vi "Compare Dependency Sets.vi"(8 "error in (no error)":errorcluster, 10 "Scanned":set{string}(c389) caption="Scanned Dependencies", 11 "Builder in":refnum<class "Builder.lvclass">) -> (0 "error out":errorcluster, 3 "Builder out":refnum<class "Builder.lvclass">)   [LabVIEW 2019, in "Builder.lvclass"]
uses:
  Builder.lvclass
  Builder.lvclass/Builder.ctl
  8787f5ba-6225-4483-b00e-ce340b9170cf.vi
  f372c00e-bb7a-4085-9e1c-f3356340c9e9.vi
  <vilib>/Utility/error.llb/Error Cluster From Error Code.vi
  <vilib>/ErrorRing/Error Ring.xnode
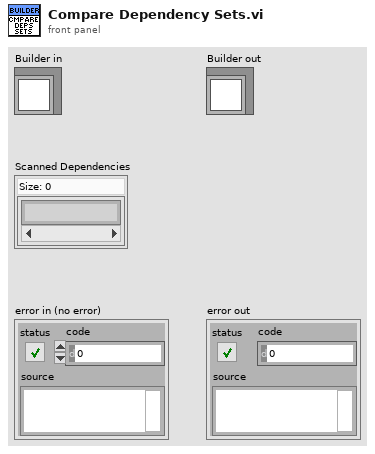
[diagram p1: front panel]
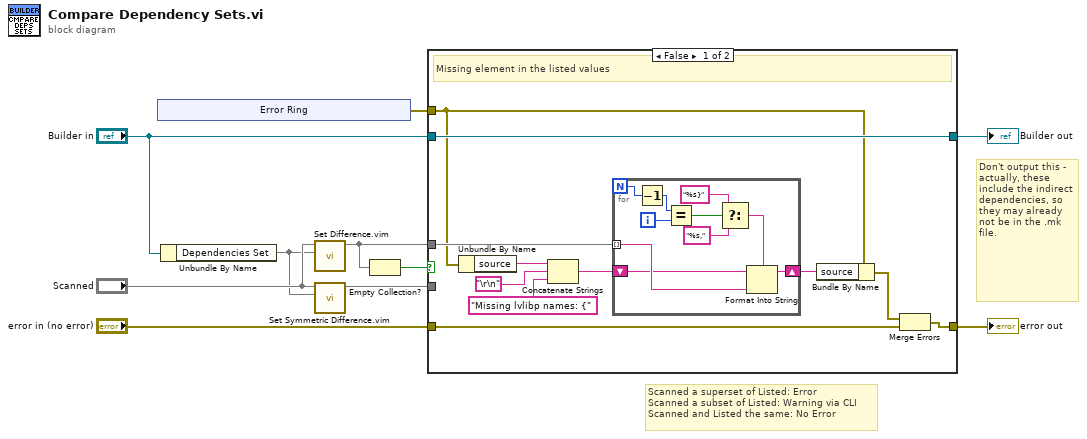
[diagram p0: block diagram]
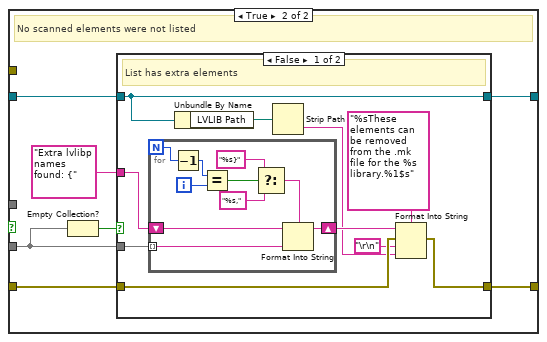
[diagram p2: hidden frame]
diagram:
  # "Don't output this - actually, these include the indirect dependencies, so they may already not be in the .mk file."
  # "Scanned a superset of Listed: Error\nScanned a subset of Listed: Warning via CLI\nScanned and Listed the same: No Error"
  n1 = xnode "Error Ring"() -> ("error out"=w1:errorcluster)
  n2 = Unbundle By Name("Builder in") -> ("Dependencies Set"=w2:set{string})
  n3 = call "Set Difference.vim"("set 2"=w2, "set 1"="Scanned") -> ("difference"=w6:set{string})  [unwired: 9 in]
  n4 = call "Set Symmetric Difference.vim"("set 2"=w2, "set 1"="Scanned") -> ("symmetric difference"=w9:set{string})  [unwired: 9 in]
  n5 = Empty Collection?(1:w6) -> (0:w4:bool)
  n6 = case shown="False" w4 {
    tunnel: w6 -> [w21 _]
    tunnel: "error in (no error)" -> [w20 w33]
    tunnel: [w19 w34] -> w8
    tunnel: w9 -> [_ w35]
    tunnel: "Builder in" -> [w18 w37]
    tunnel: [w18 w36] -> w10
    tunnel: w1 -> [w17 _]
    frame False {
      # "Missing element in the listed values"
      n7 = Unbundle By Name(w17) -> ("source"=w16:string)
      n8 = Concatenate Strings(w16, "\r\n", "Missing lvlibp names: {" ("string")) -> (w15:string)
      n9 = for {
        N -> [w28]
        tunnel: w21 -> [w31] mode=indexing
        shift-right: [w29] -> w11
        shift-left: w15 -> [w30]
        i -> [w26]
        n10 = Decrement(x=w28) -> (x-1=w27:i32)
        n11 = Equal?(x=w27, y=w26) -> (x = y?=w25:bool)
        n12 = Select(t="%s}", s=w25, f="%s,") -> (s? t:f=w22:string)
        n13 = Format Into String(format string=w22, initial string=w30, w31) -> (resulting string=w29:string)  [unwired: 1 in, 1 out]
      }
      n14 = Bundle By Name(cluster=w17, "source"=w11) -> (w12:errorcluster)
      n15 = Merge Errors(w12, w20) -> (w19:errorcluster)
    }
    frame True {
      # "No scanned elements were not listed"
      n16 = Empty Collection?(1:w35) -> (0:w38:bool)
      n17 = case shown="False" w38 {
        tunnel: w37 -> [w46 w60]
        tunnel: [w46 w60] -> w36
        tunnel: w35 -> [w47 _]
        tunnel: w33 -> [w42 w59]
        tunnel: [w43 w59] -> w34
        tunnel: "Extra lvlibp names found: {" ("string") -> [w48 _]
        frame False {
          # "List has extra elements"
          n18 = for {
            N -> [w55]
            tunnel: w47 -> [w58] mode=indexing
            shift-right: [w56] -> w44
            shift-left: w48 -> [w57]
            i -> [w53]
            n19 = Decrement(x=w55) -> (x-1=w54:i32)
            n20 = Equal?(x=w54, y=w53) -> (x = y?=w52:bool)
            n21 = Select(t="%s}", s=w52, f="%s,") -> (s? t:f=w49:string)
            n22 = Format Into String(format string=w49, initial string=w57, w58) -> (resulting string=w56:string)  [unwired: 1 in, 1 out]
          }
          n23 = Unbundle By Name(w46) -> ("LVLIB Path"=w45:path)
          n24 = Strip Path(path=w45) -> (name=w40:string)  [unwired: 1 out]
          n25 = Format Into String(format string="%sThese elements can be removed from the .mk file for the %s library.%1$s", initial string=w44, error in=w42, "\r\n", w40) -> (error out=w43:errorcluster)  [unwired: 1 out]
        }
        frame True {
          # "List matches Scanned"
        }
      }
    }
  }
  "Builder out" <- w10
  "error out" <- w8
